vi "is a.vi"(8 "error in (no error)":errorcluster, 11 "Thermometer in":refnum<class "Thermometer.lvclass">) -> (0 "error out":errorcluster, 2 "is a":string, 3 "Thermometer out":refnum<class "Thermometer.lvclass">)   [LabVIEW 2016, in "Hardware.lvlib" / "Thermometer.lvlib" / "Thermometer.lvclass"]
uses:
  <userlib>/Common Components/Hardware/Thermometer/Thermometer.lvclass
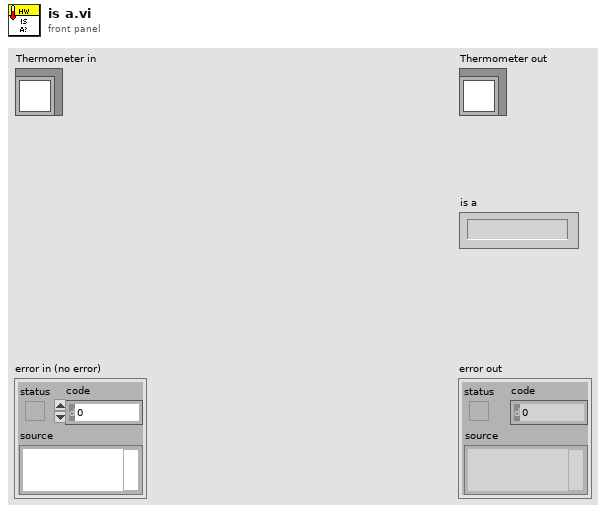
[diagram p1: front panel]
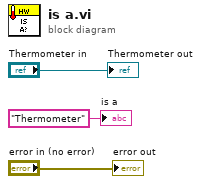
[diagram p0: block diagram]
diagram:
  "error out" <- "error in (no error)"
  "Thermometer out" <- "Thermometer in"
  "is a" <- "Thermometer" ("is a")
